vi "Converter_get_baseline_str_arr.vi"(9 "From unit #":i32, 10 "Baselines per unit in":T1, 11 "Table in":refnum<vi>) -> (3 "Baselines per unit out":string[](array[string]))   [LabVIEW 2013]
uses:
  Converter_baseline_indicator.ctl
panel:
  # "this is for use in eval formula string as replacement for variable"
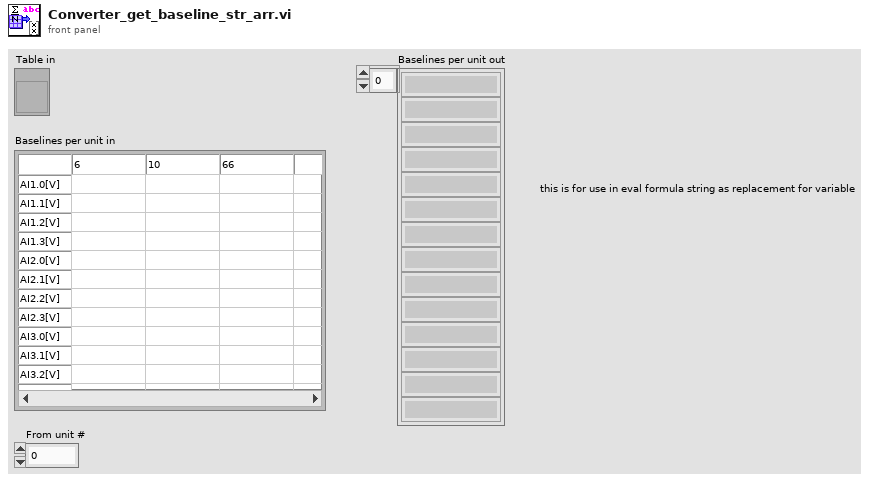
[diagram p1: front panel]
types:
  T1 = typedef "Converter_baseline_indicator.ctl" = string[][]
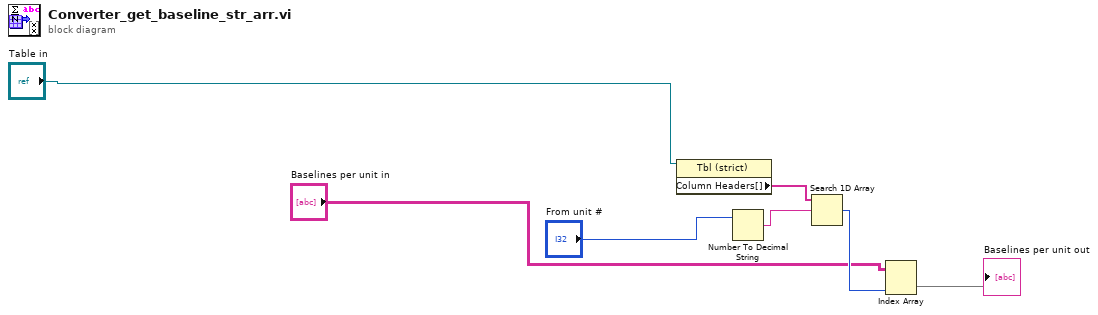
[diagram p0: block diagram]
diagram:
  n1 = property class="Tbl (strict)"(reference="Table in") -> ("Column Headers[]"=w2:string[])  [unwired: 1 in, 2 out]
  n2 = Number To Decimal String(number="From unit #") -> (decimal integer string=w3:string)  [unwired: 1 in]
  n3 = Search 1D Array(1D array=w2, element=w3) -> (index of element=w6:i32)  [unwired: 1 in]
  n4 = Index Array(array="Baselines per unit in", index (col)=w6) -> (element=→"Baselines per unit out":string[])  [unwired: 1 in]
